vi "IO_DataQ_Init.vi"(10 "Command\nList":string[](array[string])=["nop\nnop", "endo 120", "dout 56", "nop"], 11 "VISA Refnum in":refnum<visa-resource-name>="COM3") -> (0 "error out":errorcluster, 2 "Connected?":bool, 3 "VISA resource name out":refnum<visa-resource-name>="COM3")   [LabVIEW 2024]
uses:
  <vilib>/Utility/error.llb/DialogType.ctl
  <vilib>/Instr/_visa.llb/VISA Configure Serial Port (Instr).vi
panel:
  out "read buffer":string
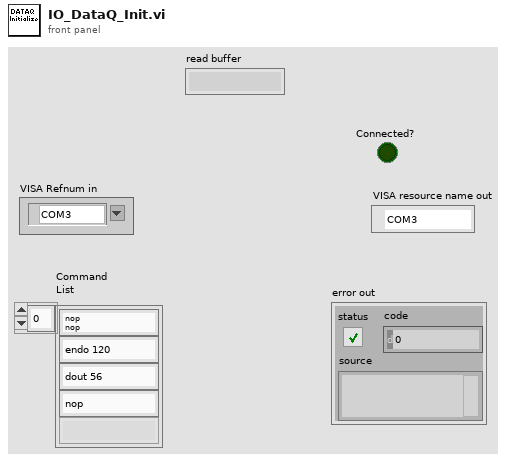
[diagram p1: front panel]
types:
  T1 = typedef "DialogType.ctl" = u16
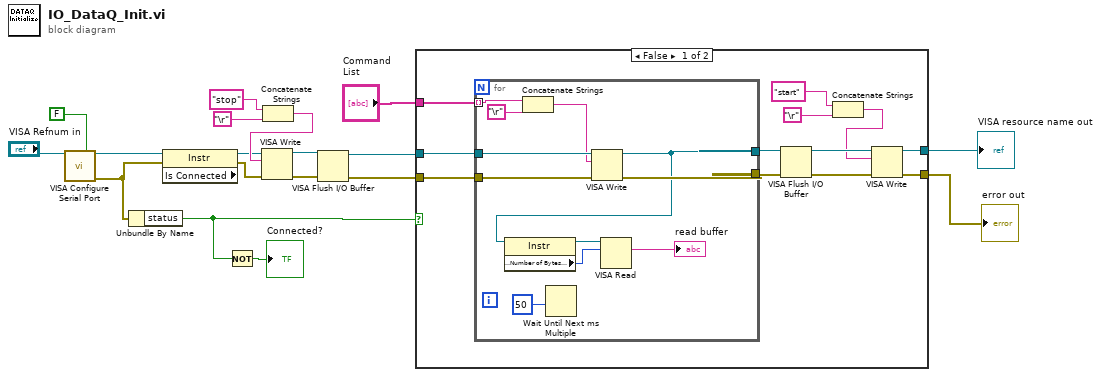
[diagram p0: block diagram]
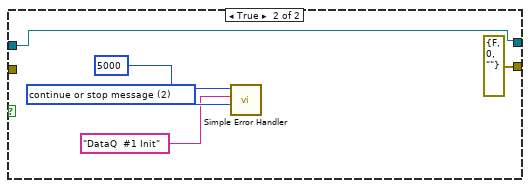
[diagram p2: hidden frame]
diagram:
  n1 = call-poly "VISA Configure Serial Port"("VISA resource name"="VISA Refnum in", "Enable Termination\nChar (T)"=FALSE) -> ("VISA resource name out"=w16:refnum<visa-resource-name>, "error out"=w12:errorcluster)  [unwired: 8 in, 4 out]
  n2 = Unbundle By Name(w12) -> ("status"=w10:bool)
  n3 = property class="Instr" props=["Is Connected"](reference=w16, error in=w12) -> (reference out=w6:refnum<visa-resource-name>, error out=w5:errorcluster)  [unwired: 1 out]
  n4 = Not(x=w10) -> (.not. x?=→"Connected?":bool)
  n5 = Concatenate Strings("stop", "\r") -> (w9:string)
  n6 = VISA Write(VISA resource name=w6, write buffer=w9, error in (no error)=w5) -> (VISA resource name out=w4:refnum<visa-resource-name>, error out=w2:errorcluster)  [unwired: 1 out]
  n7 = VISA Flush I/O Buffer(VISA resource name=w4, error in (no error)=w2) -> (VISA resource name out=w3:refnum<visa-resource-name>, error out=w1:errorcluster)  [unwired: 1 in]
  n8 = case shown="False" w10 {
    tunnel: w1 -> [w30 _]
    tunnel: w3 -> [w29 w45]
    tunnel: [w21 w45] -> w15
    tunnel: [w20 errorcluster {"status"=FALSE, "code"=0, "source"=""} ("error out")] -> w14
    tunnel: "Command\nList" -> [w19 _]
    frame False {
      n9 = for {
        tunnel: w19 -> [w38] mode=indexing
        tunnel: w29 -> [w41]
        tunnel: w30 -> [w40]
        tunnel: [w34] -> w25
        tunnel: [w35] -> w27
        n10 = Concatenate Strings(w38, "\r") -> (w36:string)
        n11 = Wait Until Next ms Multiple(millisecond multiple=u32 50 ("milliseconds to wait")) -> ()  [unwired: 1 out]
        n12 = VISA Write(VISA resource name=w41, write buffer=w36, error in (no error)=w40) -> (VISA resource name out=w34:refnum<visa-resource-name>, error out=w35:errorcluster)  [unwired: 1 out]
        n13 = property class="Instr"(reference=w34) -> (reference out=w33:refnum<visa-resource-name>, "Serial Settings:Number of Bytes at Serial Port"=w32:u32)  [unwired: 1 in, 1 out]
        n14 = VISA Read(VISA resource name=w33, byte count=w32) -> (read buffer=→"read buffer":string)  [unwired: 1 in, 3 out]
      }
      n15 = VISA Flush I/O Buffer(VISA resource name=w25, error in (no error)=w27) -> (VISA resource name out=w26:refnum<visa-resource-name>, error out=w28:errorcluster)  [unwired: 1 in]
      n16 = Concatenate Strings("start", "\r") -> (w24:string)
      n17 = VISA Write(VISA resource name=w26, write buffer=w24, error in (no error)=w28) -> (VISA resource name out=w21:refnum<visa-resource-name>, error out=w20:errorcluster)  [unwired: 1 out]
    }
    frame True {
      w44 = T1 2 items=["no dialog", "OK message", "continue or stop message", "OK message + warnings", "continue/stop + warnings"] ("type of dialog (OK msg:1)")
      n18 = call <vilib>:"Simple Error Handler.vi"("error code (no error:0)"=5000, "error source (\" \")"="DataQ  #1 Init" ("error source (\" \")"), "type of dialog (OK msg:1)"=w44) -> ()  [unwired: 2 in, 5 out]
    }
  }
  "VISA resource name out" <- w15
  "error out" <- w14
